vi "Line Wise.vi"() -> ()   [LabVIEW 2017]
uses:
  <vilib>/Utility/miscctls.llb/LVRowAndColumnTypeDef.ctl
  <vilib>/Utility/miscctls.llb/LVBoundsTypeDef.ctl
panel:
  out "COUNT":dbl
  out "DURATION":dbl
  in  "Update Shift 1 Time 3":bool
  out "COUNT":dbl
  out "DURATION":dbl
  in  "Update Shift 1 Time 2":bool
  out "COUNT":dbl
  out "DURATION":dbl
  in  "Update Shift 1 Time":bool
  # "Line Wise Live Breakdown Status"
  # "Gap Leader"
  # "Logistics"
  # "Maintenance"
  # "Quality"
  # "Production"
  # "min"
  # "min"
  # "min"
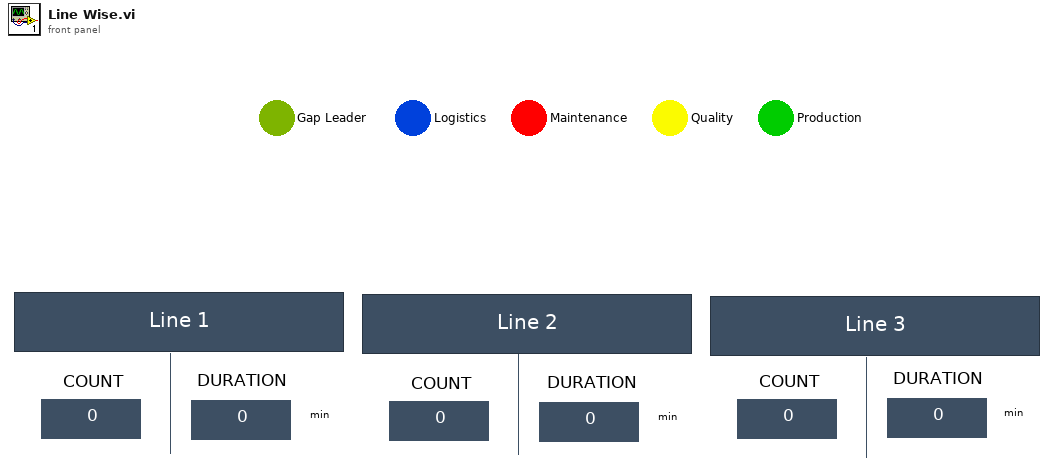
[diagram p1: front panel]
types:
  T1 = typedef "LVBoundsTypeDef.ctl" = cluster{"Width":u32, "Height":u32}
  T2 = typedef "LVRowAndColumnTypeDef.ctl" = cluster{"Row":i32, "Column":i32}
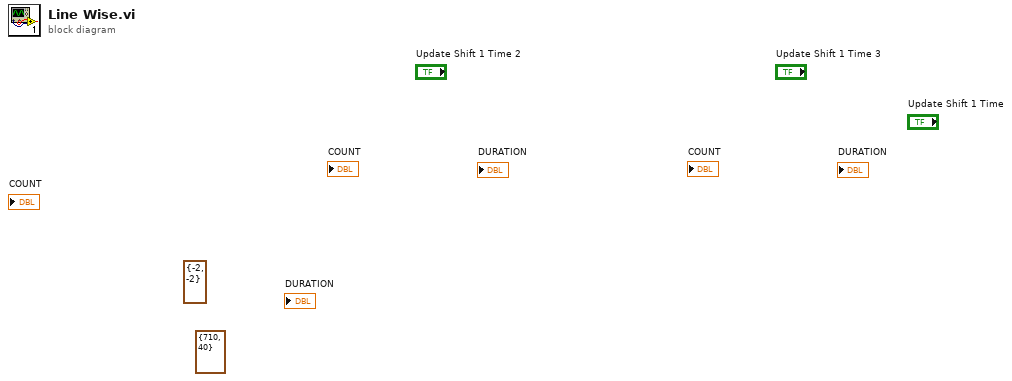
[diagram p0: block diagram]
diagram:
  (unwired) T1 {"Width"=710, "Height"=40} ("Active Cell:Cell Size")
  (unwired) T2 {"Row"=-2, "Column"=-2} ("Active Cell:Active Cell")
